vi "Flatten UIP Value.vi"(11 "UIP In":refnum<class "TipStripUIP.lvclass">) -> (0 "Error Out":errorcluster, 2 "String Value":string, 3 "UIP Out":refnum<class "TipStripUIP.lvclass">)   [LabVIEW 2015, in "TipStripUIP.lvclass"]
uses:
  TipStripUIP.lvclass
  TipStripUIP.lvclass/TipStripUIP.ctl
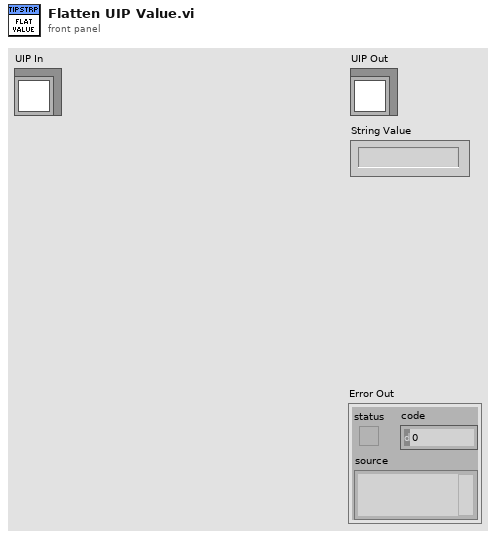
[diagram p1: front panel]
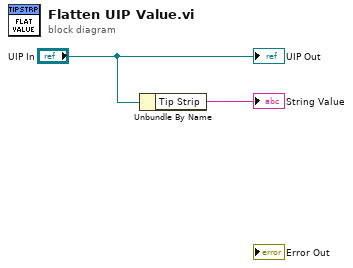
[diagram p0: block diagram]
diagram:
  n1 = Unbundle By Name("UIP In") -> ("Tip Strip"=→"String Value":string)
  "UIP Out" <- "UIP In"
